vi "ADD A Im.vi"(8 "error in (no error)":errorcluster, 10 "Im":u8 format="%04b", 11 "TD4 in":refnum<class "TD4.lvclass">) -> (0 "error out":errorcluster, 3 "TD4 out":refnum<class "TD4.lvclass">)   [LabVIEW 2025, in "TD4.lvclass"]
uses:
  TD4.lvclass
  TD4.lvclass/TD4.ctl
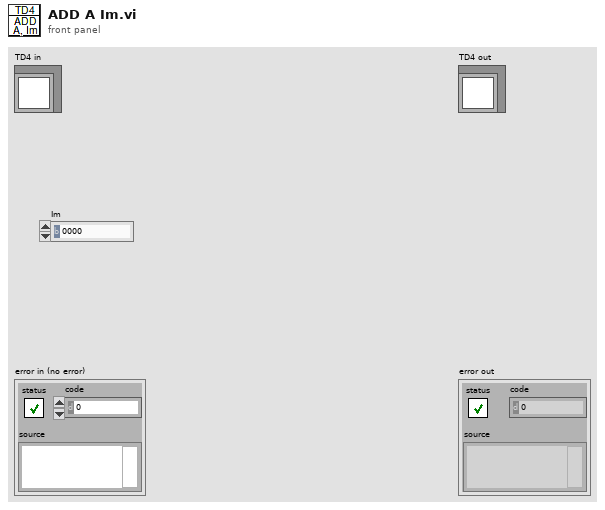
[diagram p1: front panel]
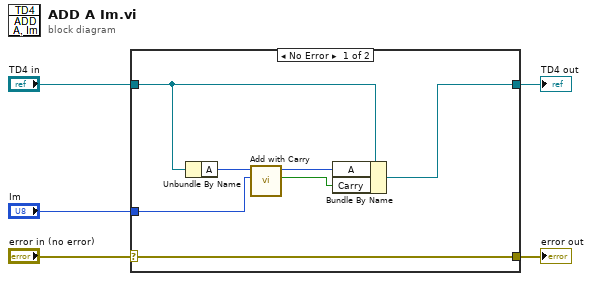
[diagram p0: block diagram]
diagram:
  n1 = case shown="No Error" "error in (no error)" {
    selector: "error in (no error)" -> [w12 w13]
    tunnel: [w12 w13] -> w4
    tunnel: [w10 w14] -> w2
    tunnel: "TD4 in" -> [w11 w14]
    tunnel: "Im" -> [w8 _]
    frame No Error {
      n2 = Unbundle By Name(w11) -> ("A"=w9:u8)
      n3 = call "Add with Carry.vi"("Input 2"=w8, "Input 1"=w9) -> ("Carry"=w6:bool, "Output"=w7:u8)  [unwired: 8 in]
      n4 = Bundle By Name(cluster=w11, "A"=w7, "Carry"=w6) -> (w10:refnum<class "TD4.lvclass">)
    }
    frame Error {
    }
  }
  "error out" <- w4
  "TD4 out" <- w2
